vi "Test Enter.vi"() -> ()   [LabVIEW 2020]
panel:
  in  "Points Settings":T1(array[cluster]) caption="Set Measurement Point"
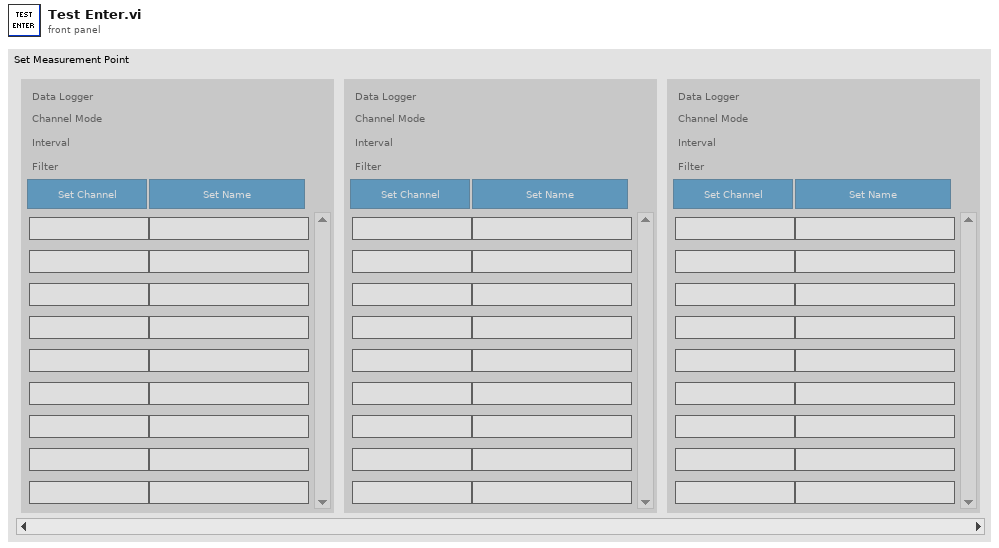
[diagram p1: front panel]
types:
  T1 = cluster{"Data Logger":string, "Channel Mode":string, "Interval":string, "Filter":string, "Channel Set":bool, "Name Set":bool, "Points":cluster{"Channel":string, "Name":string}[]}[]
  T2 = cluster{" Key":u8, "Action":enum16{"Press", "Up", "Down"}, "Delay (ms)":u32}[]
  T3 = typedef "eventvkey.ctl" = enum16{"ASCII", "Enter", "Return", "Shift", "Ctrl", "Alt", "Cmd", "Opt", "Caps", "NumLock", "Clear", "Break", "Up", "Down", "Left", "Right", "Insert", "Delete", "Home", "End", "PageUp", "PageDown", "Escape", "Help", "Pause", "ScrollLock", "F1", "F2", "F3", "F4", "F5", "F6", "F7", "F8", "F9", "F10", "F11", "F12", "F13", "F14", "F15", "F16", "F17", "F18", "F19", "F20", "F21", "F22", "F23", "F24", "Play", "VolumeUp", "VolumeDown", "Mute", "Two Byte Char"}
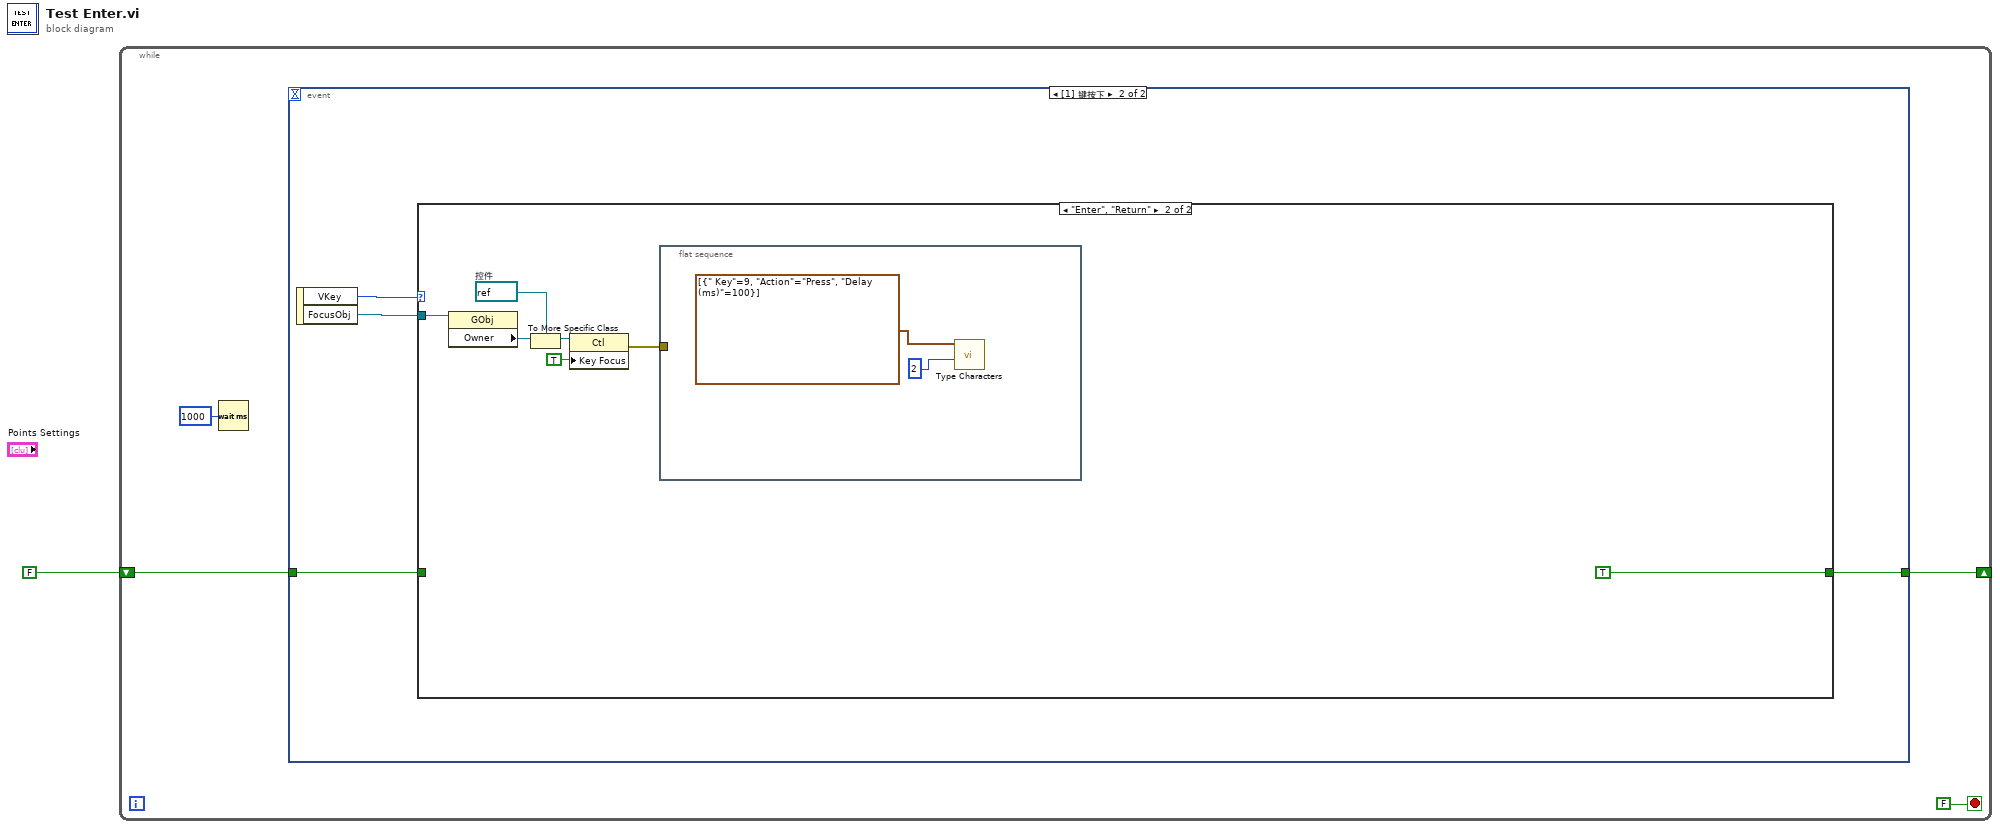
[diagram p0: block diagram]
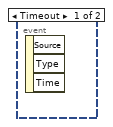
[diagram p2: hidden frame]
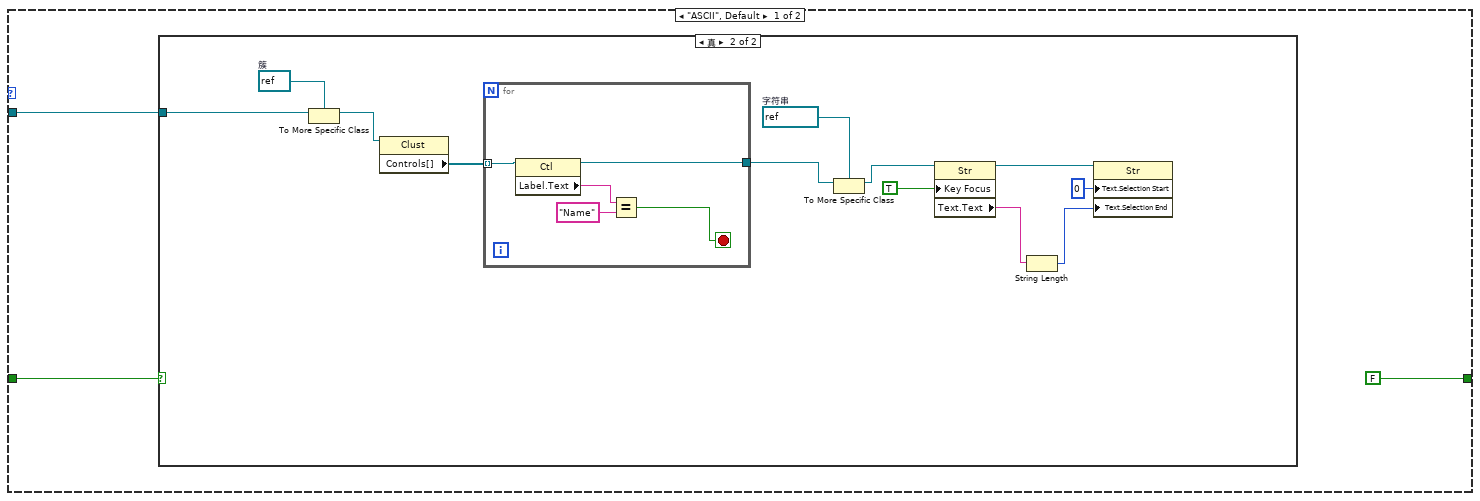
[diagram p3: hidden frame]
diagram:
  n1 = while {
    shift-right: [w3] -> _
    shift-left: FALSE -> [w4]
    stop <- FALSE stop-if-true
    n2 = Wait (ms)(milliseconds to wait=u32 1000) -> ()  [unwired: 1 out]
    n3 = event shown="[1] 键按下" {
      selector: _ -> [_ _]
      dyn-events: _ -> [_ _]
      timeout: _ -> [_ _]
      tunnel: w4 -> [_ w7]
      tunnel: [_ w6] -> w3
      event Timeout {
        n4 = event-data() -> ()  [unwired: 1 in, 3 out]
      }
      event Key Down {
        n5 = event-data() -> ("VKey"=w8:T3, "FocusObj"=w9:refnum<vi>)  [unwired: 1 in]
        n6 = case shown="\"Enter\", \"Return\"" w8 {
          tunnel: w9 -> [w12 w36]
          tunnel: w7 -> [w11 _]
          tunnel: [FALSE TRUE ("键选中")] -> w6
          frame "ASCII", Default {
            n7 = case shown="真" w11 {
              tunnel: w12 -> [_ w24]
              frame False {
              }
              frame True {
                w18 = refnum<vi> refnum  # 字符串
                w23 = refnum<vi> refnum  # 簇
                n8 = To More Specific Class(target class=w23, reference=w24) -> (specific class reference=w22:refnum<vi>)  [unwired: 1 in, 1 out]
                n9 = property class="Clust"(reference=w22) -> ("Controls[]"=w21:refnum<vi>[])  [unwired: 1 in, 2 out]
                n10 = for {
                  tunnel: w21 -> [w29] mode=indexing
                  tunnel: [w25] -> w19
                  stop <- w26 stop-if-true
                  n11 = property class="Ctl"(reference=w29) -> (reference out=w25:refnum<vi>, "Label.Text"=w28:string)  [unwired: 1 in, 1 out]
                  n12 = Equal?(x=w28, y="Name") -> (x = y?=w26:bool)
                }
                n13 = To More Specific Class(target class=w18, reference=w19) -> (specific class reference=w17:refnum<vi>)  [unwired: 1 in, 1 out]
                n14 = property class="Str"(reference=w17, "Key Focus"=TRUE ("键选中")) -> (reference out=w16:refnum<vi>, "Text.Text"=w14:string)  [unwired: 1 in, 1 out]
                n15 = String Length(string=w14) -> (length=w13:i32)
                n16 = property class="Str"(reference=w16, "Text.Selection Start"=u32 0 ("文本.选择区域:起始"), "Text.Selection End"=w13) -> ()  [unwired: 1 in, 2 out]
              }
            }
          }
          frame "Enter", "Return" {
            w35 = refnum<vi> refnum  # 控件
            n17 = property class="GObj"(reference=w36) -> ("Owner"=w34:refnum<vi>)  [unwired: 1 in, 2 out]
            n18 = To More Specific Class(target class=w35, reference=w34) -> (specific class reference=w33:refnum<vi>)  [unwired: 1 in, 1 out]
            n19 = property class="Ctl"(reference=w33, "Key Focus"=TRUE ("键选中")) -> (error out=w31:errorcluster)  [unwired: 1 in, 1 out]
            n20 = flat-sequence {
              tunnel: w31 -> [_]
              frame #0 {
                n21 = call "Type Characters.vi"("Length of Key Press (ms)"=u32 2, "Key Array"=T2 [{" Key"=9, "Action"=enum."Press", "Delay (ms)"=100}] ("Cluster")) -> ()  [unwired: 10 in]
              }
            }
          }
        }
      }
    }
  }
